vi "pathSmoothToDestArray.vi"(9 "Robot":refnum<class "Robot.lvclass">, 10 "last_path_smooth":dbl[][](array[numeric]), 11 "path_smooth":dbl[][](array[numeric])) -> (2 "new_path_smooth?":bool, 3 "dest_array":T1(array[cluster]))   [LabVIEW 2023, in "Game.lvclass"]
uses:
  Game.lvclass
  Robot_class/Robot.lvclass
  Robot_class/Robot.lvclass/Robot.ctl
  <vilib>/Analysis/_algsub.llb/Real Vector Norm.vi
  Robot_class/Read dest_x.vi
  Robot_class/Read dest_y.vi
  Robot_class/Read dest_orientation.vi
  Robot_class/Read dest_vel.vi
  <vilib>/Analysis/NI_AALPro.lvlib
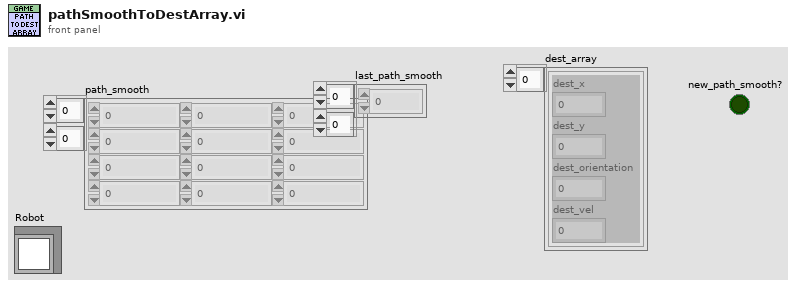
[diagram p1: front panel]
types:
  T1 = cluster{"dest_x":dbl, "dest_y":dbl, "dest_orientation":dbl, "dest_vel":dbl}[]
  T2 = cluster{"dest_x":dbl, "dest_y":dbl, "dest_orientation":dbl, "dest_vel":dbl}
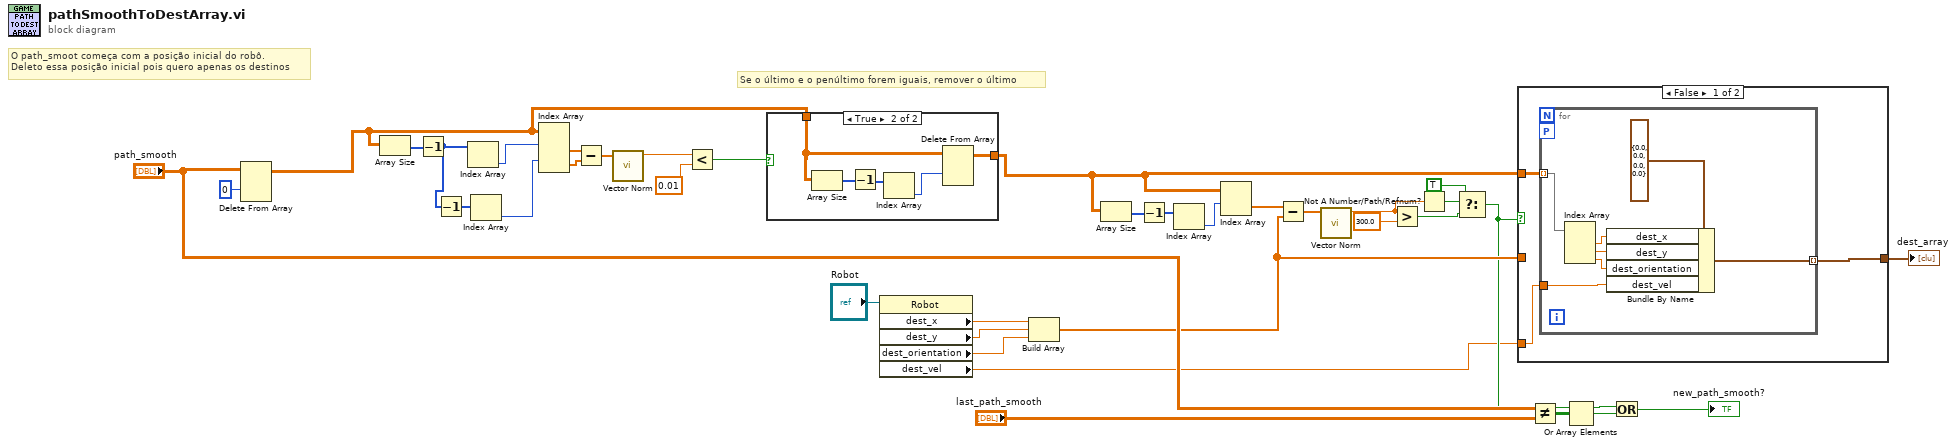
[diagram p0: block diagram]
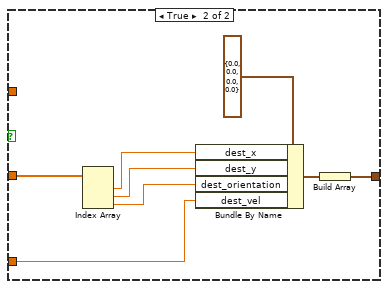
[diagram p3: hidden frame]
diagram:
  # "Se o último e o penúltimo forem iguais, remover o último"
  # "O path_smoot começa com a posição inicial do robô.\nDeleto essa posição inicial pois quero apenas os destinos"
  n1 = Delete From Array(array="path_smooth", index (row)=0) -> (array with subset deleted=w14:dbl[][])  [unwired: 2 in, 1 out]
  n2 = Array Size(array=w14) -> (size(s)=w19:i32[])
  n3 = Decrement(x=w19) -> (x-1=w18:i32[])
  n4 = Decrement(x=w18) -> (x-1=w17:i32[])
  n5 = Index Array(array=w18) -> (element=w16:i32)  [unwired: 1 in]
  n6 = Index Array(array=w17) -> (element=w15:i32)  [unwired: 1 in]
  n7 = Index Array(array=w14, index (row) #1=w16, index (row) #2=w15) -> (element #1=w12:dbl[], element #2=w11:dbl[])  [unwired: 2 in]
  n8 = Subtract(x=w12, y=w11) -> (x-y=w10:dbl[])
  n9 = call-poly <vilib>:"Vector Norm.vi"("Input Vector"=w10) -> ("norm"=w9:dbl)  [unwired: 9 in, 1 out]
  n10 = Less?(x=w9, y=0.01) -> (x < y?=w7:bool)
  n11 = case shown="True" w7 {
    tunnel: w14 -> [w38 w43]
    tunnel: [w38 w39] -> w13
    frame False {
    }
    frame True {
      n12 = Array Size(array=w43) -> (size(s)=w42:i32[])
      n13 = Decrement(x=w42) -> (x-1=w41:i32[])
      n14 = Index Array(array=w41) -> (element=w40:i32)  [unwired: 1 in]
      n15 = Delete From Array(array=w43, index (row)=w40) -> (array with subset deleted=w39:dbl[][])  [unwired: 2 in, 1 out]
    }
  }
  n16 = property class="Robot"(reference="Robot") -> ("dest_x"=w23:dbl, "dest_y"=w22:dbl, "dest_orientation"=w21:dbl, "dest_vel"=w1:dbl)  [unwired: 1 in, 2 out]
  n17 = Build Array(w23, w22, w21) -> (w20:dbl[])
  n18 = Array Size(array=w13) -> (size(s)=w32:i32[])
  n19 = Decrement(x=w32) -> (x-1=w31:i32[])
  n20 = Index Array(array=w31) -> (element=w30:i32)  [unwired: 1 in]
  n21 = Index Array(array=w13, index (row)=w30) -> (element=w29:dbl[])  [unwired: 1 in]
  n22 = Subtract(x=w29, y=w20) -> (x-y=w28:dbl[])
  n23 = call-poly <vilib>:"Vector Norm.vi"("Input Vector"=w28) -> ("norm"=w6:dbl)  [unwired: 9 in, 1 out]
  n24 = Greater?(x=w6, y=300.0) -> (0:w4:bool)
  n25 = Not A Number/Path/Refnum?(number/path/refnum=w6) -> (NaN/Path/Refnum?=w5:bool)
  n26 = Select(t=TRUE, s=w5, f=w4) -> (s? t:f=w2:bool)
  n27 = case shown="False" w2 {
    tunnel: [w46 w55] -> w37
    tunnel: w13 -> [w45 _]
    tunnel: w20 -> [_ w60]
    tunnel: w1 -> [w44 w54]
    frame False {
      n28 = for {
        tunnel: w45 -> [w52] mode=indexing
        tunnel: [w48] -> w46 mode=indexing
        tunnel: w44 -> [w47]
        workers-P: _ -> [_]
        n29 = Index Array(array=w52) -> (element #1=w51:dbl, element #2=w50:dbl, element #3=w49:dbl)  [unwired: 3 in]
        n30 = Bundle By Name(cluster=T2 {"dest_x"=0.0, "dest_y"=0.0, "dest_orientation"=0.0, "dest_vel"=0.0} ("Dest_array"), "dest_x"=w51, "dest_y"=w50, "dest_orientation"=w49, "dest_vel"=w47) -> (w48:T2)
      }
    }
    frame True {
      n31 = Index Array(array=w60) -> (element #1=w59:dbl, element #2=w58:dbl, element #3=w57:dbl)  [unwired: 3 in]
      n32 = Bundle By Name(cluster=T2 {"dest_x"=0.0, "dest_y"=0.0, "dest_orientation"=0.0, "dest_vel"=0.0} ("Dest_array"), "dest_x"=w59, "dest_y"=w58, "dest_orientation"=w57, "dest_vel"=w54) -> (w56:T2)
      n33 = Build Array(w56) -> (w55:T1)
    }
  }
  "dest_array" <- w37
  n34 = Not Equal?(x="path_smooth", y="last_path_smooth") -> (x != y?=w33:bool[][])
  n35 = Or Array Elements(Boolean array=w33) -> (logical OR=w26:bool)
  n36 = Or(x=w2, y=w26) -> (x .or. y?=→"new_path_smooth?":bool)
